vi "FileAdministrotar.vi"() -> ()   [LabVIEW 2018]
uses:
  Subvi/Global.vi
panel:
  out "字符串":string
  in  "退出":bool
  in  "删除":bool
  in  "Test Item":i32(listbox)
  out "filenames":string[](array[string])
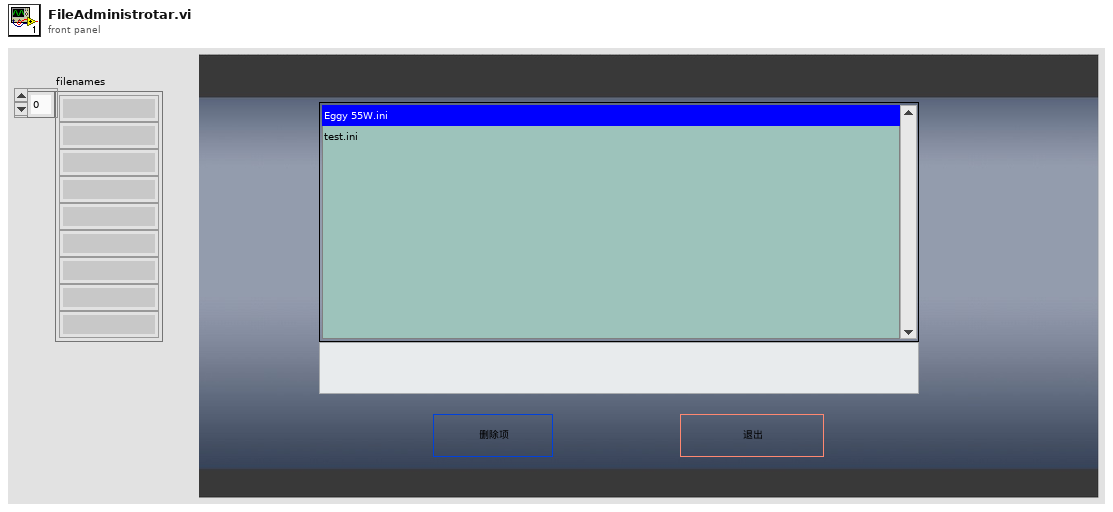
[diagram p1: front panel]
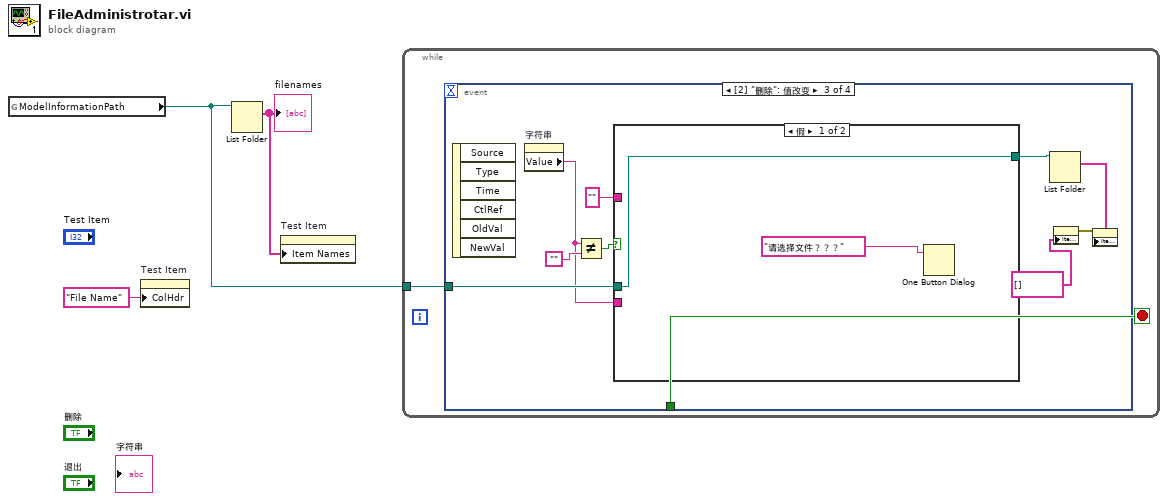
[diagram p0: block diagram]
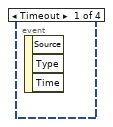
[diagram p2: hidden frame]
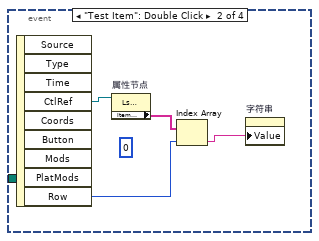
[diagram p3: hidden frame]
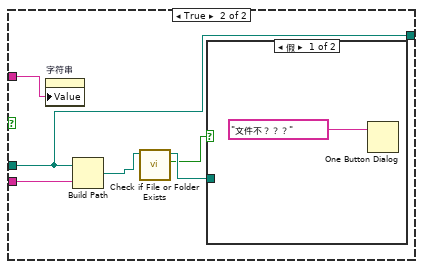
[diagram p4: hidden frame]
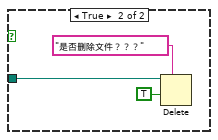
[diagram p5: hidden frame]
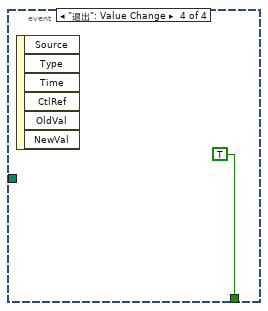
[diagram p6: hidden frame]
diagram:
  n1 = global read "Global.vi" "ModelInformationPath"() -> (w1:path)
  n2 = property on="Test Item" class="LstBox (严格)"("ColHdr"="File Name" ("列首字符串")) -> ()  [unwired: 2 in, 2 out]
  n3 = List Folder(path=w1) -> (filenames=w2:string[])  [unwired: 3 in, 3 out]
  "filenames" <- w2
  n4 = property on="Test Item" class="LstBox (严格)"("Item Names"=w2) -> ()  [unwired: 2 in, 2 out]
  n5 = while {
    tunnel: w1 -> [w4]
    stop <- w5 stop-if-true
    n6 = event shown="[2] \"删除\": 值改变" {
      selector: _ -> [_ _ _ _]
      dyn-events: _ -> [_ _ _ _]
      timeout: _ -> [_ _ _ _]
      tunnel: [_ _ _ TRUE] -> w5
      tunnel: w4 -> [_ _ w16 _]
      event Timeout {
        n7 = event-data() -> ()  [unwired: 1 in, 3 out]
      }
      event "Test Item": Double Click {
        (unwired) 0 ("禁用的索引 (列)")
        n8 = event-data() -> ("CtlRef"=w9:refnum<vi>, "Row"=w7:i32)  [unwired: 1 in, 7 out]
        n9 = property on="属性节点" class="LstBox (严格)"(reference=w9) -> ("Item Names"=w8:string[])  [unwired: 1 in, 2 out]
        n10 = Index Array(array=w8, index=w7) -> (element=w6:string)
        n11 = property on="字符串" class="Str"("Value"=w6) -> ()  [unwired: 2 in, 2 out]
      }
      event "删除": Value Change {
        n12 = event-data() -> ()  [unwired: 1 in, 6 out]
        n13 = property on="字符串" class="Str"() -> ("Value"=w15:string)  [unwired: 2 in, 2 out]
        n14 = Not Equal?(x=w15, y="") -> (x != y?=w18:bool)
        n15 = case shown="假" w18 {
          tunnel: w16 -> [w19 w21]
          tunnel: w15 -> [_ w26]
          tunnel: "" -> [_ w22]
          tunnel: [w19 w21] -> w12
          frame False {
            n16 = One Button Dialog(message="请选择文件？？？" ("对话框窗口（删除）")) -> ()  [unwired: 1 in, 1 out]
          }
          frame True {
            n17 = property on="字符串" class="Str"("Value"=w22) -> ()  [unwired: 2 in, 2 out]
            n18 = Build Path(base path=w21, name or relative path=w26) -> (appended path=w25:path)
            n19 = call <vilib>:"Check if File or Folder Exists.vi"("path"=w25) -> ("file or folder exists?"=w23:bool, "dup path"=w24:path)  [unwired: 8 in, 1 out]
            n20 = case shown="假" w23 {
              tunnel: w24 -> [_ w30]
              frame False {
                n21 = One Button Dialog(message="文件不？？？" ("对话框窗口（删除）")) -> ()  [unwired: 1 in, 1 out]
              }
              frame True {
                n22 = Delete(prompt (Delete)="是否删除文件？？？" ("对话框窗口（删除）"), path (use dialog)=w30, confirm (F)=TRUE ("确认(F)")) -> ()  [unwired: 2 in, 3 out]
              }
            }
          }
        }
        n23 = List Folder(path=w12) -> (filenames=w13:string[])  [unwired: 3 in, 3 out]
        n24 = property on="Test Item" class="LstBox (严格)"("Item Names"=string[] []) -> (error out=w11:errorcluster)  [unwired: 2 in, 1 out]
        n25 = property on="Test Item" class="LstBox (严格)"(error in=w11, "Item Names"=w13) -> ()  [unwired: 1 in, 2 out]
      }
      event "退出": Value Change {
        n26 = event-data() -> ()  [unwired: 1 in, 6 out]
      }
    }
  }
